vi "User_Login.vi"() -> ()   [LabVIEW 2020]
uses:
  <vilib>/Utility/cursorutil.llb/Set Cursor (Icon Pict).vi
panel:
  in  "Remember User Name":bool caption="记住用户名"
  in  "Remember Passwrod":bool caption="记住密码"
  in  "Register":bool
  in  "Login":bool
  in  "User_Password":string caption="密    码"
  in  "User_Name":string caption="用户名"
  # "登录系统"
  # "@Agaido再度科技"
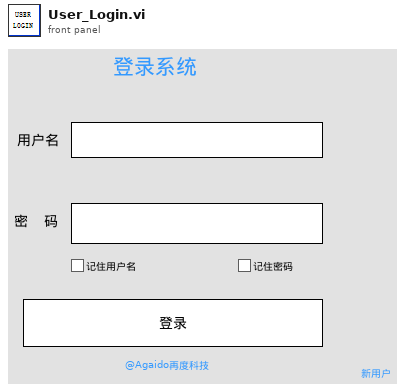
[diagram p1: front panel]
types:
  T1 = enum32{"Invalid", "Standard", "Closed", "Hidden", "Minimized", "Maximized"}
  T2 = typedef "User_Info.ctl" = cluster{"Name":string, "Password":string, "User_Right":u16, "Debuger?":bool, "Manager?":bool, "User_Remember_Name":bool, "User_Remember_PW":bool, "User_Right_String":string, "Null?":bool, "Language":string}
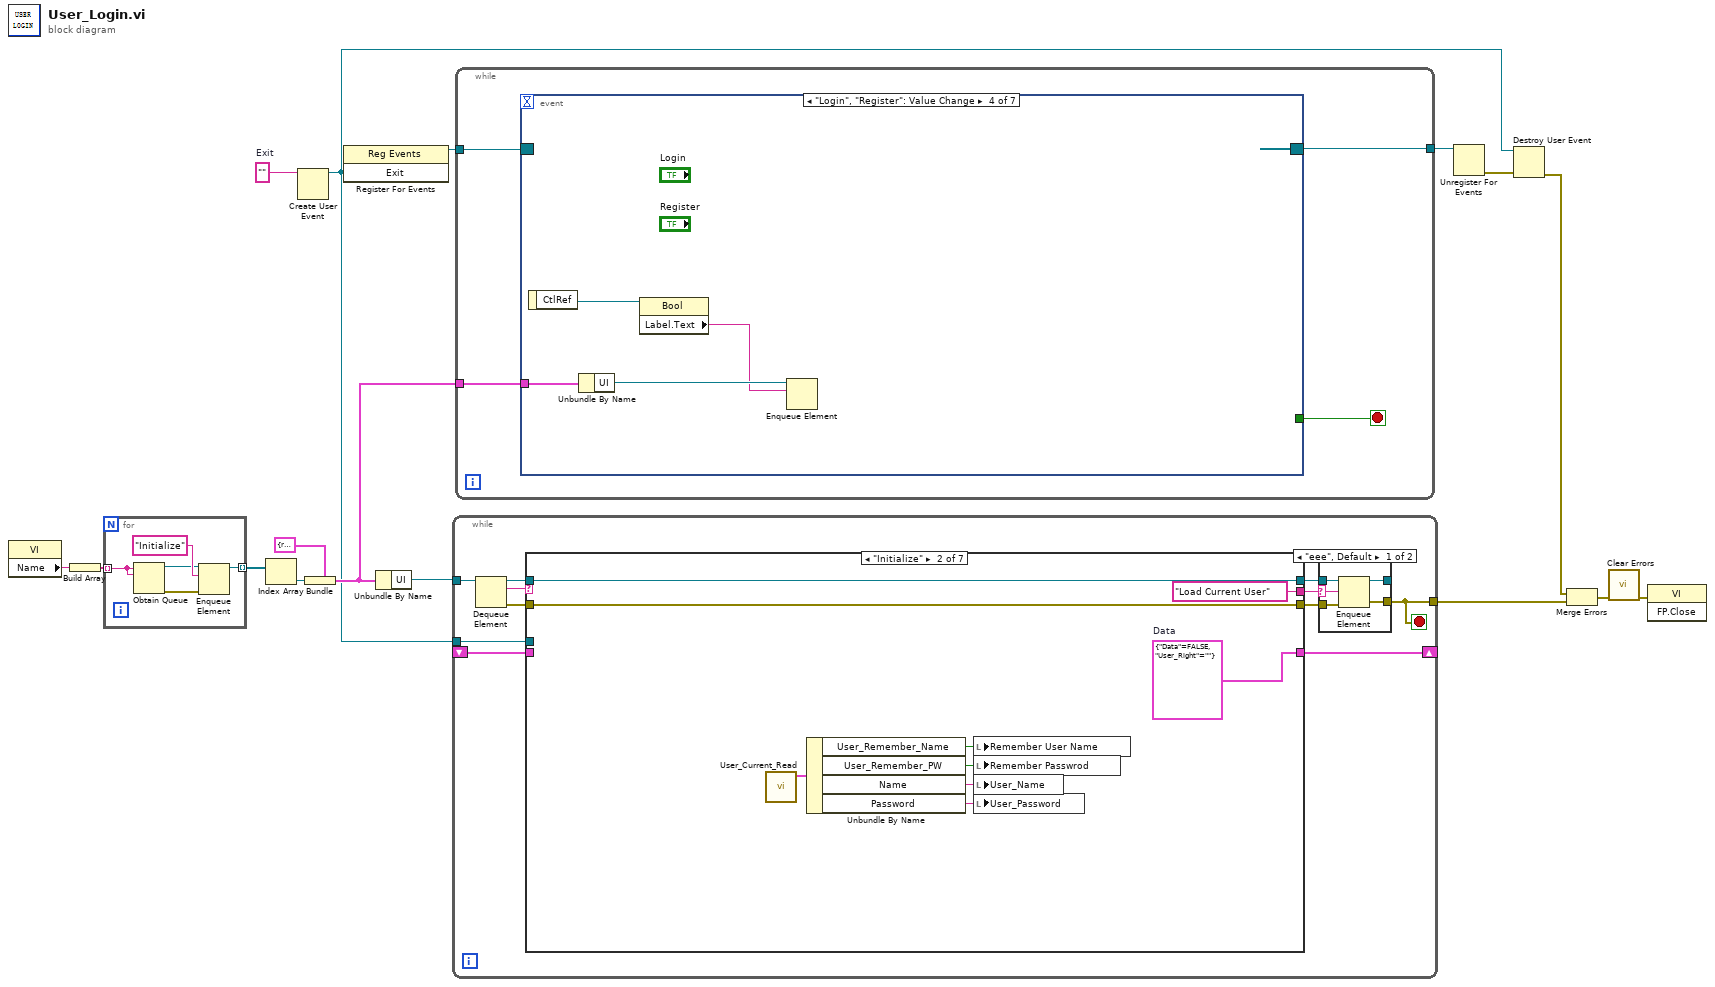
[diagram p0: block diagram]
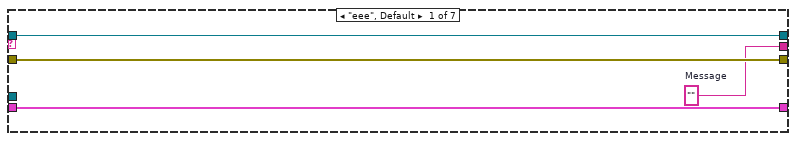
[diagram p3: hidden frame]
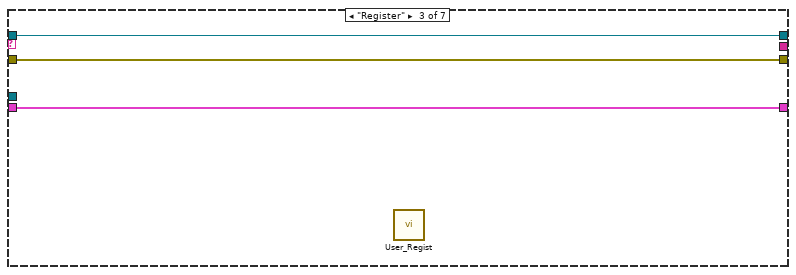
[diagram p4: hidden frame]
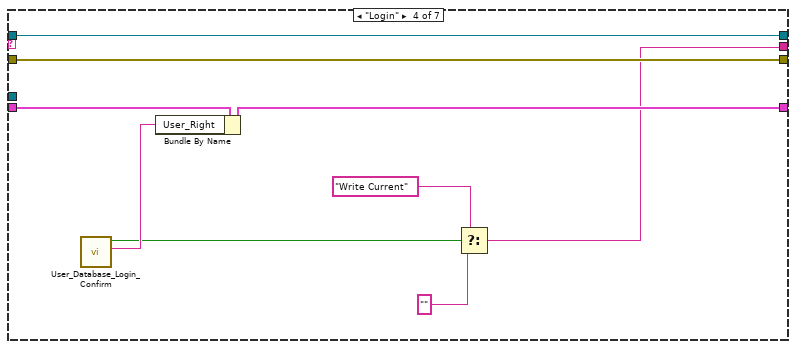
[diagram p5: hidden frame]
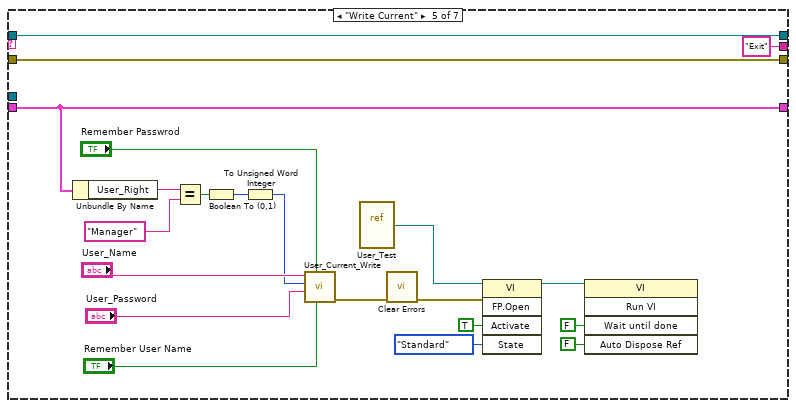
[diagram p6: hidden frame]
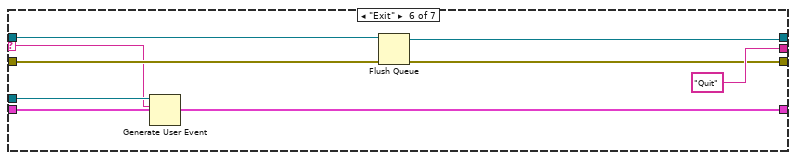
[diagram p7: hidden frame]
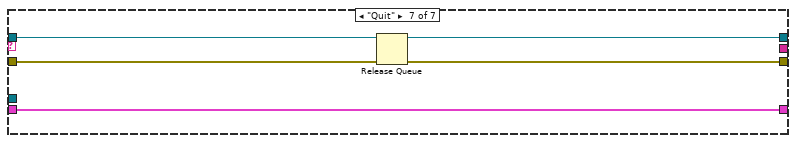
[diagram p8: hidden frame]
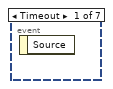
[diagram p9: hidden frame]
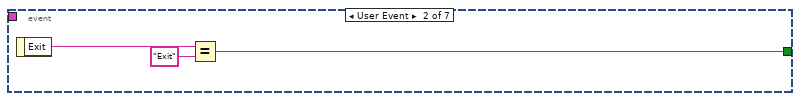
[diagram p10: hidden frame]
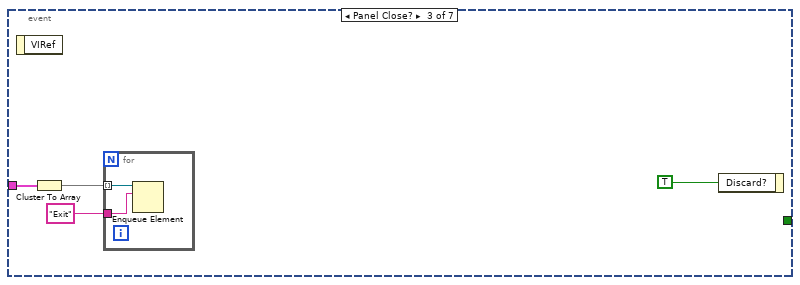
[diagram p11: hidden frame]
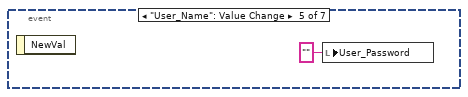
[diagram p12: hidden frame]
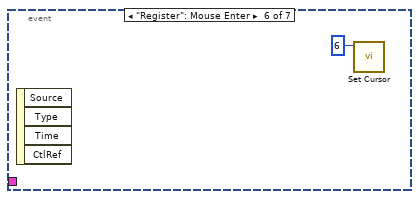
[diagram p13: hidden frame]
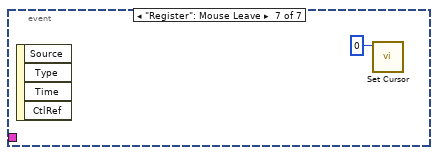
[diagram p14: hidden frame]
diagram:
  w2 = ""  # Exit
  n1 = property class="VI"() -> ("Name"=w12:string)  [unwired: 2 in, 2 out]
  n2 = Build Array(w12) -> (w13:string[])
  n3 = for {
    tunnel: w13 -> [w17] mode=indexing
    tunnel: [w18] -> w7 mode=indexing
    n4 = Obtain Queue(name (unnamed)=w17, element data type=w17) -> (queue out=w20:refnum<queue>, error out=w19:errorcluster)  [unwired: 3 in, 1 out]
    n5 = Enqueue Element(queue=w20, element="Initialize" ("元素"), error in (no error)=w19) -> (queue out=w18:refnum<queue>)  [unwired: 1 in, 2 out]
  }
  n6 = Index Array(array=w7) -> (element=w10:refnum<queue>)  [unwired: 1 in]
  n7 = Create User Event(user event datatype=w2) -> (user event=w6:refnum<user-event>)  [unwired: 1 in, 1 out]
  n8 = Bundle(cluster=cluster{"UI":refnum<queue>} {"UI"=refnum}, "UI"=w10) -> (w11:cluster{"UI":refnum<queue>})
  n9 = register-events(w6) -> (reference out=w3:refnum<event-registration>)  [unwired: 2 in, 1 out]
  n10 = Unbundle By Name(w11) -> ("UI"=w8:refnum<queue>)
  n11 = while {
    tunnel: w8 -> [w32]
    tunnel: [w22] -> w15
    shift-right: [w26] -> _
    shift-left: _ -> [w25]
    tunnel: w6 -> [w24]
    stop <- w22 stop-if-true
    n12 = Dequeue Element(queue=w32) -> (queue out=w31:refnum<queue>, element=w23:string, error out=w28:errorcluster)  [unwired: 2 in, 1 out]
    n13 = case shown="\"Initialize\"" w23 {
      selector: w23 -> [_ _ _ _ _ w86 _]
      tunnel: w31 -> [w43 w52 w55 w64 w85 w91 w97]
      tunnel: [w43 w52 w55 w64 w85 w90 w97] -> w30
      tunnel: [w42 w51 w54 w63 w84 w89 w94] -> w29
      tunnel: w28 -> [w42 w51 w54 w63 w84 w88 w96]
      tunnel: [w41 "Load Current User" ("Message") _ w56 "Exit" ("Message") "Quit" ("Message") _] -> w27
      tunnel: [w40 w50 w53 w61 w77 w93 w95] -> w26
      tunnel: w25 -> [w40 _ w53 w62 w77 w93 w95]
      tunnel: w24 -> [_ _ _ _ _ w87 _]
      frame "eee", Default {
        w41 = ""  # Message
      }
      frame "Initialize" {
        w50 = cluster{"Data":bool, "User_Right":string} {"Data"=FALSE, "User_Right"=""}  # Data
        n14 = call "User_Current_Read.vi"() -> ("User_Info"=w48:T2)  [unwired: 10 in, 1 out]
        n15 = Unbundle By Name(w48) -> ("User_Remember_Name"=w47:bool, "User_Remember_PW"=w46:bool, "Name"=w45:string, "Password"=w44:string)
        n16 = local write "Remember User Name"(w47) -> ()
        n17 = local write "Remember Passwrod"(w46) -> ()
        n18 = local write "User_Name"(w45) -> ()
        n19 = local write "User_Password"(w44) -> ()
      }
      frame "Register" {
        n20 = call "User_Regist.vi"() -> ()  [unwired: 12 in]
      }
      frame "Login" {
        n21 = call "User_Database_Login_Confirm.vi"() -> ("User_Right"=w60:string, "OK"=w59:bool)  [unwired: 9 in, 1 out]
        n22 = Bundle By Name(cluster=w62, "User_Right"=w60) -> (w61:cluster{"Data":bool, "User_Right":string})
        n23 = Select(t="Write Current", s=w59, f="") -> (s? t:f=w56:string)
      }
      frame "Write Current" {
        n24 = Unbundle By Name(w77) -> ("User_Right"=w81:string)
        n25 = Equal?(x=w81, y="Manager") -> (x = y?=w79:bool)
        n26 = Boolean To (0,1)(Boolean=w79) -> (0, 1=w78:i16)
        n27 = To Unsigned Word Integer(number=w78) -> (unsigned 16bit integer=w76:u16)
        n28 = call "User_Current_Write.vi"("User_Remember_Name"="Remember User Name", "User_Remember_PW"="Remember Passwrod", "Password"="User_Password", "User_Right"=w76, "Name"="User_Name") -> ("error out"=w66:errorcluster)  [unwired: 6 in]
        n29 = vi-ref "User_Test.vi"() -> (w71:refnum<vi>)
        n30 = call <vilib>:"Clear Errors.vi"("error in (no error)"=w66) -> ("error out"=w65:errorcluster)  [unwired: 5 in, 1 out]
        n31 = invoke class="VI" method="FP.Open"(reference=w71, error in=w65, "Activate"=TRUE ("激活？"), "State"=T1."Standard" ("状态")) -> (reference out=w72:refnum<vi>)  [unwired: 1 in, 4 out]
        n32 = invoke class="VI" method="Run VI"(reference=w72, "Wait until done"=FALSE ("结束前等待"), "Auto Dispose Ref"=FALSE ("自动销毁引用")) -> ()  [unwired: 2 in, 5 out]
      }
      frame "Exit" {
        n33 = Generate User Event(user event=w87, event data cluster=w86) -> ()  [unwired: 2 in, 2 out]
        n34 = Flush Queue(queue=w91, error in (no error)=w88) -> (queue out=w90:refnum<queue>, error out=w89:errorcluster)  [unwired: 1 out]
      }
      frame "Quit" {
        n35 = Release Queue(queue=w97, error in (no error)=w96) -> (error out=w94:errorcluster)  [unwired: 1 in, 2 out]
      }
    }
    n36 = case shown="\"eee\", Default" w27 {
      selector: w27 -> [w33 _]
      tunnel: w30 -> [w37 w39]
      tunnel: w29 -> [w36 w38]
      tunnel: [w35 w38] -> w22
      tunnel: [w34 w39] -> _
      frame "eee", Default {
        n37 = Enqueue Element(queue=w37, element=w33, error in (no error)=w36) -> (queue out=w34:refnum<queue>, error out=w35:errorcluster)  [unwired: 1 in, 1 out]
      }
      frame "" {
      }
    }
  }
  n38 = while {
    tunnel: w3 -> [w100]
    tunnel: [w99] -> w5
    tunnel: w11 -> [w98]
    stop <- w101 stop-if-true
    n39 = event shown="[3] \"Login\", \"Register\": Value Change" {
      selector: w100 -> [_ _ _ _ _ _ _]
      dyn-events: [_ _ _ _ _ _ _] -> w99
      timeout: _ -> [_ _ _ _ _ _ _]
      tunnel: [_ w103 _ _ _ _ _] -> w101
      tunnel: w98 -> [_ _ w107 w114 _ _ _]
      event Timeout {
        n40 = event-data() -> ()  [unwired: 1 in, 1 out]
      }
      event User Event {
        n41 = event-data() -> ("Exit"=w104:string)  [unwired: 1 in]
        n42 = Equal?(x=w104, y="Exit") -> (x = y?=w103:bool)
      }
      event Panel Close? {
        n43 = event-data() -> ()  [unwired: 1 in, 1 out]
        n44 = Cluster To Array(cluster=w107) -> (array=w106:refnum<queue>[])
        n45 = for {
          tunnel: w106 -> [w110] mode=indexing
          tunnel: "Exit" ("元素") -> [w109]
          n46 = Enqueue Element(queue=w110, element=w109) -> ()  [unwired: 2 in, 3 out]
        }
        n47 = event-data("Discard?"=TRUE ("放弃？")) -> ()  [unwired: 1 in, 1 out]
      }
      event "Login", "Register": Value Change {
        n48 = event-data() -> ("CtlRef"=w112:refnum<vi>)  [unwired: 1 in]
        n49 = Unbundle By Name(w114) -> ("UI"=w113:refnum<queue>)
        n50 = property class="Bool"(reference=w112) -> ("Label.Text"=w111:string)  [unwired: 1 in, 2 out]
        n51 = Enqueue Element(queue=w113, element=w111) -> ()  [unwired: 2 in, 3 out]
      }
      event "User_Name": Value Change {
        n52 = event-data() -> ()  [unwired: 1 in, 1 out]
        n53 = local write "User_Password"("" ("User_Password")) -> ()
      }
      event "Register": Mouse Enter {
        n54 = event-data() -> ()  [unwired: 1 in, 4 out]
        n55 = call-poly <vilib>:"Set Cursor.vi"("icon"=u16 6) -> ()  [unwired: 9 in, 2 out]
      }
      event "Register": Mouse Leave {
        n56 = event-data() -> ()  [unwired: 1 in, 4 out]
        n57 = call-poly <vilib>:"Set Cursor.vi"("icon"=u16 0) -> ()  [unwired: 9 in, 2 out]
      }
    }
  }
  n58 = Unregister For Events(event registration refnum=w5) -> (error out=w4:errorcluster)  [unwired: 1 in]
  n59 = Destroy User Event(user event=w6, error in=w4) -> (error out=w14:errorcluster)
  n60 = Merge Errors(w14, w15) -> (w16:errorcluster)
  n61 = call <vilib>:"Clear Errors.vi"("error in (no error)"=w16) -> ("error out"=w1:errorcluster)  [unwired: 5 in, 1 out]
  n62 = invoke class="VI" method="FP.Close"(error in=w1) -> ()  [unwired: 2 in, 3 out]
